vi "SaveRealData.vi"(10 "2D data":string[][](array[string]), 11 "ProductID":string) -> ()   [LabVIEW 2017]
uses:
  Ctrls/PathChoose.ctl
  <vilib>/Utility/file.llb/Write Delimited Spreadsheet (string).vi
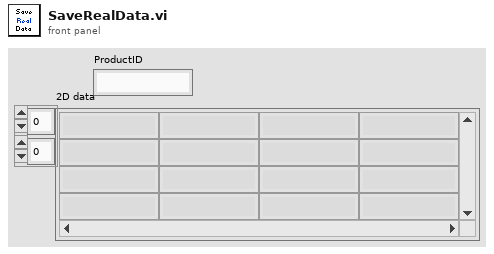
[diagram p1: front panel]
types:
  T1 = typedef "PathChoose.ctl" = enum16{"OperatorLog", "AutoRunLog", "AlmLog", "TestData", "AllTestData"}
  T2 = enum16{"open", "replace", "create", "open or create", "replace or create", "replace or create with confirmation"}
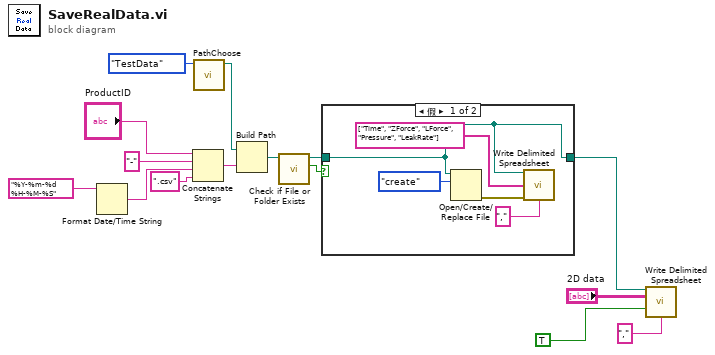
[diagram p0: block diagram]
diagram:
  n1 = Format Date/Time String(time format string (%c)="%Y-%m-%d %H-%M-%S") -> (date/time string=w5:string)  [unwired: 2 in]
  n2 = Concatenate Strings("ProductID", "-" ("string"), w5, ".csv" ("string")) -> (w7:string)
  n3 = call "PathChoose.vi"(11:PathChoose."TestData") -> ("Path_Out"=w12:path)  [unwired: 10 in]
  n4 = Build Path(base path=w12, name or relative path=w7) -> (appended path=w8:path)
  n5 = call <vilib>:"Check if File or Folder Exists.vi"("path"=w8) -> ("file or folder exists?"=w10:bool, "dup path"=w9:path)  [unwired: 8 in, 1 out]
  n6 = case shown="假" w10 {
    tunnel: w9 -> [w18 w21]
    tunnel: [w18 w21] -> w15
    frame False {
      n7 = Open/Create/Replace File(file path (use dialog)=w18, operation (0:open)=T2."create") -> (error out=w17:errorcluster)  [unwired: 4 in, 2 out]
      n8 = call-poly <vilib>:"Write Delimited Spreadsheet.vi"("file path (dialog if empty)"=w18, "1D data"=string[] ["Time", "ZForce", "LForce", "Pressure", "LeakRate"], "error in (no error)"=w17, "delimiter (\\t)"="," ("delimiter (\\t)")) -> ()  [unwired: 10 in, 2 out]
    }
    frame True {
    }
  }
  n9 = call-poly <vilib>:"Write Delimited Spreadsheet.vi"("file path (dialog if empty)"=w15, "2D data"="2D data", "append to file? (new file:F)"=TRUE, "delimiter (\\t)"="," ("delimiter (\\t)")) -> ()  [unwired: 10 in, 2 out]
